vi "Strings and Values.vi"(8 "error in (no error)":errorcluster, 11 "Remote Systems in":refnum<class "Remote Systems.lvclass">) -> (0 "error out":errorcluster, 2 "Strings And Values []":T1, 3 "Remote Systems out":refnum<class "Remote Systems.lvclass">)   [LabVIEW 2020, in "Remote Systems.lvclass"]
uses:
  Remote Systems.lvclass
  <vilib>/Utility/miscctls.llb/LVComboBoxStrsAndValuesArrayTypeDef.ctl
  Remote Systems.lvclass/Remote Systems.ctl
  <vilib>/nisyscfg/Close (System).vi
  <vilib>/regexp/Match Regular Expression.xnode
  <vilib>/nisyscfg/nisyscfg.lvlib
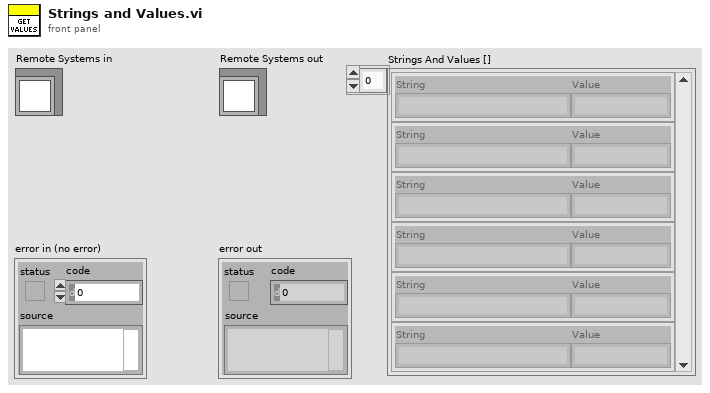
[diagram p1: front panel]
types:
  T1 = typedef "LVComboBoxStrsAndValuesArrayTypeDef.ctl" = cluster{"String":string, "Value":string}[]
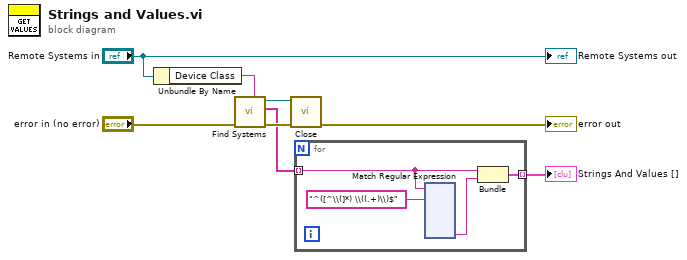
[diagram p0: block diagram]
diagram:
  n1 = Unbundle By Name("Remote Systems in") -> ("Device Class"=w4:string)
  n2 = call <vilib>:"Find Systems.vi"("Device Class"=w4, "error in (no error)"="error in (no error)") -> ("error out"=w7:errorcluster, "Detected Systems"=w2:string[], "Session out"=w8:refnum<k21>)  [unwired: 7 in]
  n3 = call-poly <vilib>:"Close.vi"("error in (no error)"=w7, "Session in"=w8) -> ("error out"=→"error out":errorcluster)  [unwired: 9 in]
  n4 = for {
    tunnel: w2 -> [w11] mode=indexing
    tunnel: [w9] -> w1 mode=indexing
    n5 = xnode "Match Regular Expression"("input string"=w11, "regular expression"="^([^\\(]*) \\((.+)\\)$") -> ("submatch 2"=w10:string)  [unwired: 4 in, 6 out]
    n6 = Bundle("String"=w11, "submatch 2"=w10) -> (w9:cluster{"String":string, "submatch 2":string})  [unwired: 1 in]
  }
  "Strings And Values []" <- w1
  "Remote Systems out" <- "Remote Systems in"
